vi "Load Config.vi"(8 "error in (no error)":errorcluster, 11 "GUI Manager Module in":refnum<class "GUI Manager Module.lvclass">) -> (0 "error out":errorcluster, 3 "GUI Manager Module out":refnum<class "GUI Manager Module.lvclass">)   [LabVIEW 2020, in "VolatusGUI.lvlib" / "GUI Manager Module.lvclass"]
uses:
  GUI Manager Module.lvclass
  Volatus/Module/Module.lvclass/Module.ctl
  VolatusConfig/VolatusConfigElement/VolatusConfigElement.lvclass/VolatusConfigElement.ctl
  GUI Manager Module.lvclass/GUI Manager Module.ctl
  Volatus/Module/Config.vi
  VolatusConfig/VolatusConfigElement/Lookup Child by Name.vi
  VolatusConfig/VolatusConfigElement/Element.vi
  lv-cdm/CDM-Config/Config Element/Lookup Child by Name.vi
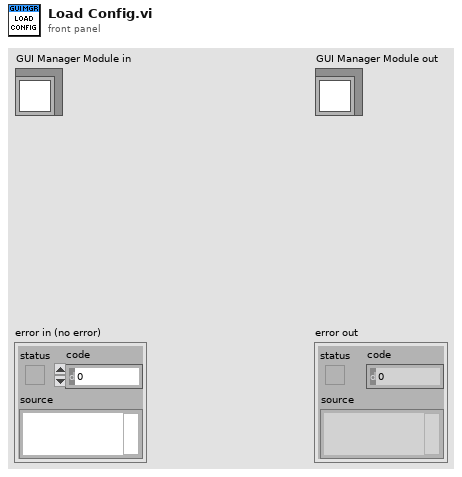
[diagram p1: front panel]
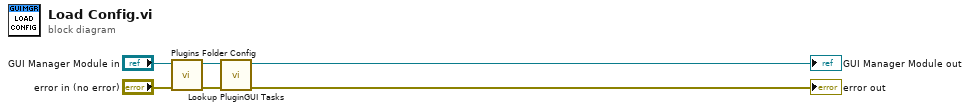
[diagram p0: block diagram]
diagram:
  n1 = call "Plugins Folder Config.vi"("error in (no error)"="error in (no error)", "GUI Manager Module in"="GUI Manager Module in") -> ("error out"=w3:errorcluster, "GUI Manager Module out"=w4:refnum<class "GUI Manager Module.lvclass">)  [unwired: 8 in]
  n2 = call "Lookup PluginGUI Tasks.vi"("error in (no error)"=w3, "GUI Manager Module in"=w4) -> ("error out"=→"error out":errorcluster, "GUI Manager Module out"=→"GUI Manager Module out":refnum<class "GUI Manager Module.lvclass">)  [unwired: 8 in]
